vi "Memory.Pointer.Read.Subset.Safe (1D U8).vi"(8 "error in (no error)":errorcluster, 9 "offset (0)":u64 format="%d bytes", 10 "length":u64=18446744073709551615 format="%d bytes", 11 "Pointer in":refnum<class "Memory.Pointer.lvclass">) -> (0 "error out":errorcluster, 1 "offset dup":u64 format="%d bytes", 2 "buffer out":u8[](array[numeric]) format="%02x", 3 "Pointer out":refnum<class "Memory.Pointer.lvclass">)   [LabVIEW 2016, in "LabVIEW Memory Manager.lvlib" / "Memory.Pointer.lvclass"]
uses:
  Memory.Pointer.lvclass
  Memory.Pointer.lvclass/Memory.Pointer.ctl
  Memory.Pointer.Read.Subset.In Place.Unsafe (1D U8).vi
  Memory.Pointer.Offset to Address.vi
  Memory.Pointer.Offset to Address.Unsafe.vi
  Accessors/Memory.Pointer.Get Address.vi
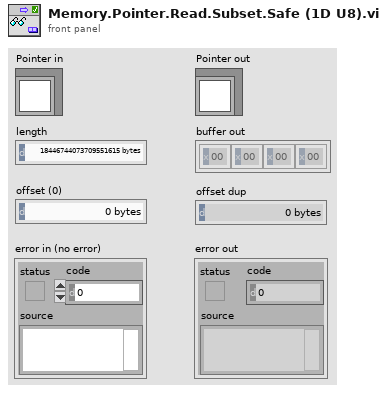
[diagram p1: front panel]
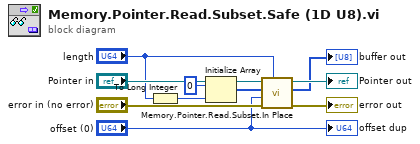
[diagram p0: block diagram]
diagram:
  n1 = To Long Integer(number="length") -> (32bit integer=w3:i32)
  n2 = Initialize Array(u8 0 ("element"), w3) -> (w2:u8[])
  n3 = call-poly "Memory.Pointer.Read.Subset.In Place.vi"("length"="length", "error in (no error)"="error in (no error)", "offset (0)"="offset (0)", "buffer in"=w2, "Pointer in"="Pointer in") -> ("error out"=→"error out":errorcluster, "buffer out"=→"buffer out":u8[], "Pointer out"=→"Pointer out":refnum<class "Memory.Pointer.lvclass">)  [unwired: 3 in, 1 out]
  "offset dup" <- "offset (0)"
